vi "HeadPrint API.vi"(6 "Timeout (ms)":u32=30000, 8 "error in (no error)":errorcluster, 10 "HeadPrint Data":T1={"PrintImageFile"="", "PrintPass"=0, "EncoderSource"="", "PrintGoSource"="", "Head"=enum."1"}, 11 "TopLevel in":refnum<class "TopLevel.lvclass">) -> (0 "error out":errorcluster, 3 "TopLevel out":refnum<class "TopLevel.lvclass">)   [LabVIEW 2022 SP3, in "TopLevel.lvclass"]
uses:
  TopLevel.lvclass
  Typedefs/HeadPrintData--Cluster.ctl
  Typedefs/PrinterHeads--Enum.ctl
  Typedefs/API Command Cluster.ctl
  Typedefs/API Command Enum.ctl
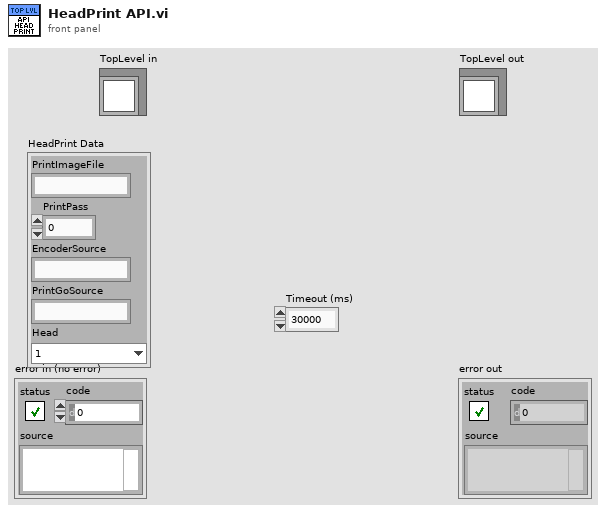
[diagram p1: front panel]
types:
  T1 = typedef "TopLevel.lvclass/HeadPrintData--Cluster.ctl" = cluster{"PrintImageFile":string, "PrintPass":u8, "EncoderSource":string, "PrintGoSource":string, "Head":T2}
  T2 = typedef "PrinterHeads--Enum.ctl" = enum16{"-1", "1", "2", "3", "4", "5", "6"}
  T3 = typedef "TopLevel.lvclass/API Command Enum.ctl" = enum16{"Execute Printer Commands", "Pre Purge", "Enable Ink Ch-1", "Enable Ink Ch-2", "Enable Ink Ch-3", "Enable Ink Ch-4", "Enable Ink Ch-5", "Enable Ink Ch-6", "Disable Ink Ch-1", "Disable Ink Ch-2", "Disable Ink Ch-3", "Disable Ink Ch-4", "Disable Ink Ch-5", "Disable Ink Ch-6", "ExecuteIdlePrintCycle", "StopIdlePrintCycle", "Abort", "LoadDLP2GUIConfig", "SaveDLP2GUIConfig", "PrimingMode", "SetHeadTemperature", "EnableHead", "EnableHeadHeat", "SetSystemMode", "HeadPrint", "AbortAll", "Send Printer String", "WriteInitXML"}
  T4 = typedef "TopLevel.lvclass/API Command Cluster.ctl" = cluster{"Command":T3, "Arguments":string, "Data":variant}
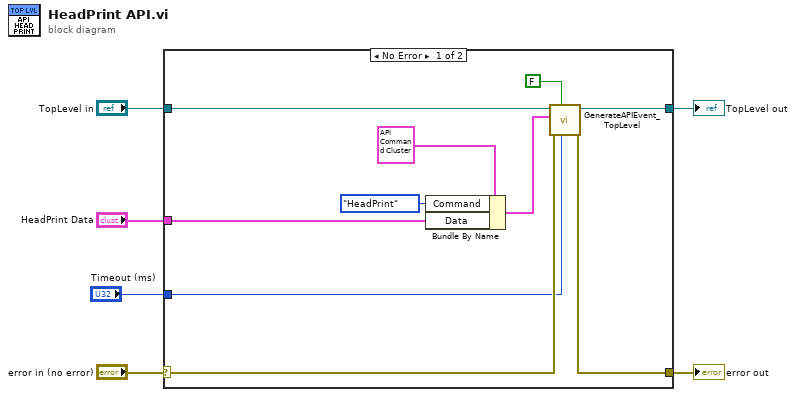
[diagram p0: block diagram]
diagram:
  n1 = case shown="No Error" "error in (no error)" {
    selector: "error in (no error)" -> [w14 w18]
    tunnel: [w13 w18] -> w5
    tunnel: [w16 w17] -> w3
    tunnel: "TopLevel in" -> [w15 w17]
    tunnel: "HeadPrint Data" -> [w8 _]
    tunnel: "Timeout (ms)" -> [w7 _]
    frame No Error {
      n2 = Bundle By Name(cluster=T4 {"Command"=enum."Execute Printer Commands", "Arguments"="", "Data"=variant} ("API Command Cluster"), "Command"=API_Command_Enum."HeadPrint", "Data"=w8) -> (w10:T4)
      n3 = call-dynamic "GenerateAPIEvent_TopLevel.vi"("Timeout (ms)"=w7, "Wait (F)"=FALSE, "error in (no error)"=w14, "API Command Cluster"=w10, "TopLevel in"=w15) -> ("error out"=w13:errorcluster, "TopLevel out"=w16:refnum<class "TopLevel.lvclass">)  [unwired: 5 in]
    }
    frame Error {
    }
  }
  "error out" <- w5
  "TopLevel out" <- w3
